vi "Read Teller.vi"(11 "Terminate Msg in":refnum<class "Terminate Msg.lvclass">) -> (2 "Teller":refnum<class "Teller.lvclass">)   [LabVIEW 2025, in "jettl.lvlib" / "Terminate Msg.lvlib" / "Terminate Msg.lvclass"]
uses:
  Terminate Msg.lvclass
  Terminate Msg.lvclass/Terminate Msg.ctl
  Teller/Teller/Teller.lvclass
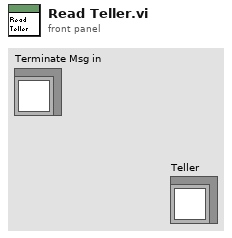
[diagram p1: front panel]
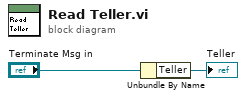
[diagram p0: block diagram]
diagram:
  n1 = Unbundle By Name("Terminate Msg in") -> ("Teller"=→"Teller":refnum<class "Teller.lvclass">)
